vi "Periodic Tasks.vi"(8 "error in":errorcluster) -> ()   [LabVIEW 2016]
doc: "This VI runs in parallel to other tasks. It can contain as many user-defined periodic loops as you need. These can carry out PID or other sorts of timed response."
uses:
  <vilib>/Rock Robotics/WPI/Utilities/WPI_GetSetVariantRefNum.vi
  <vilib>/Rock Robotics/Network Tables/NT Write Number.vi
  <vilib>/Instr/_visa.llb/VISA Configure Serial Port (Instr).vi
  Systems/Global 1.vi
  Global 2.vi
panel:
  in  "Gyro Reset":bool
  out "Angle":dbl
  in  "Reset Drive":bool
  out "Waveform Chart":dbl(graph)
  out "PSI":dbl=101.0986199
  out "Shoot 0":dbl format="%#_13g"
  out "Shoot 1":dbl format="%#_13g"
  out "read buffer":string="B:2,X:203.00"
  in  "Search_Params":string[](array[string])=["B", "X", "Y", "W1", "H1", "W2", "H2"]
  out "Last Complete Message":string="B:2,X:203.00,Y:125.00,W1:11,H1:27,W2:8,H2:25"
  out "length":i32=44
  in  "off set":dbl format="%#_13g"
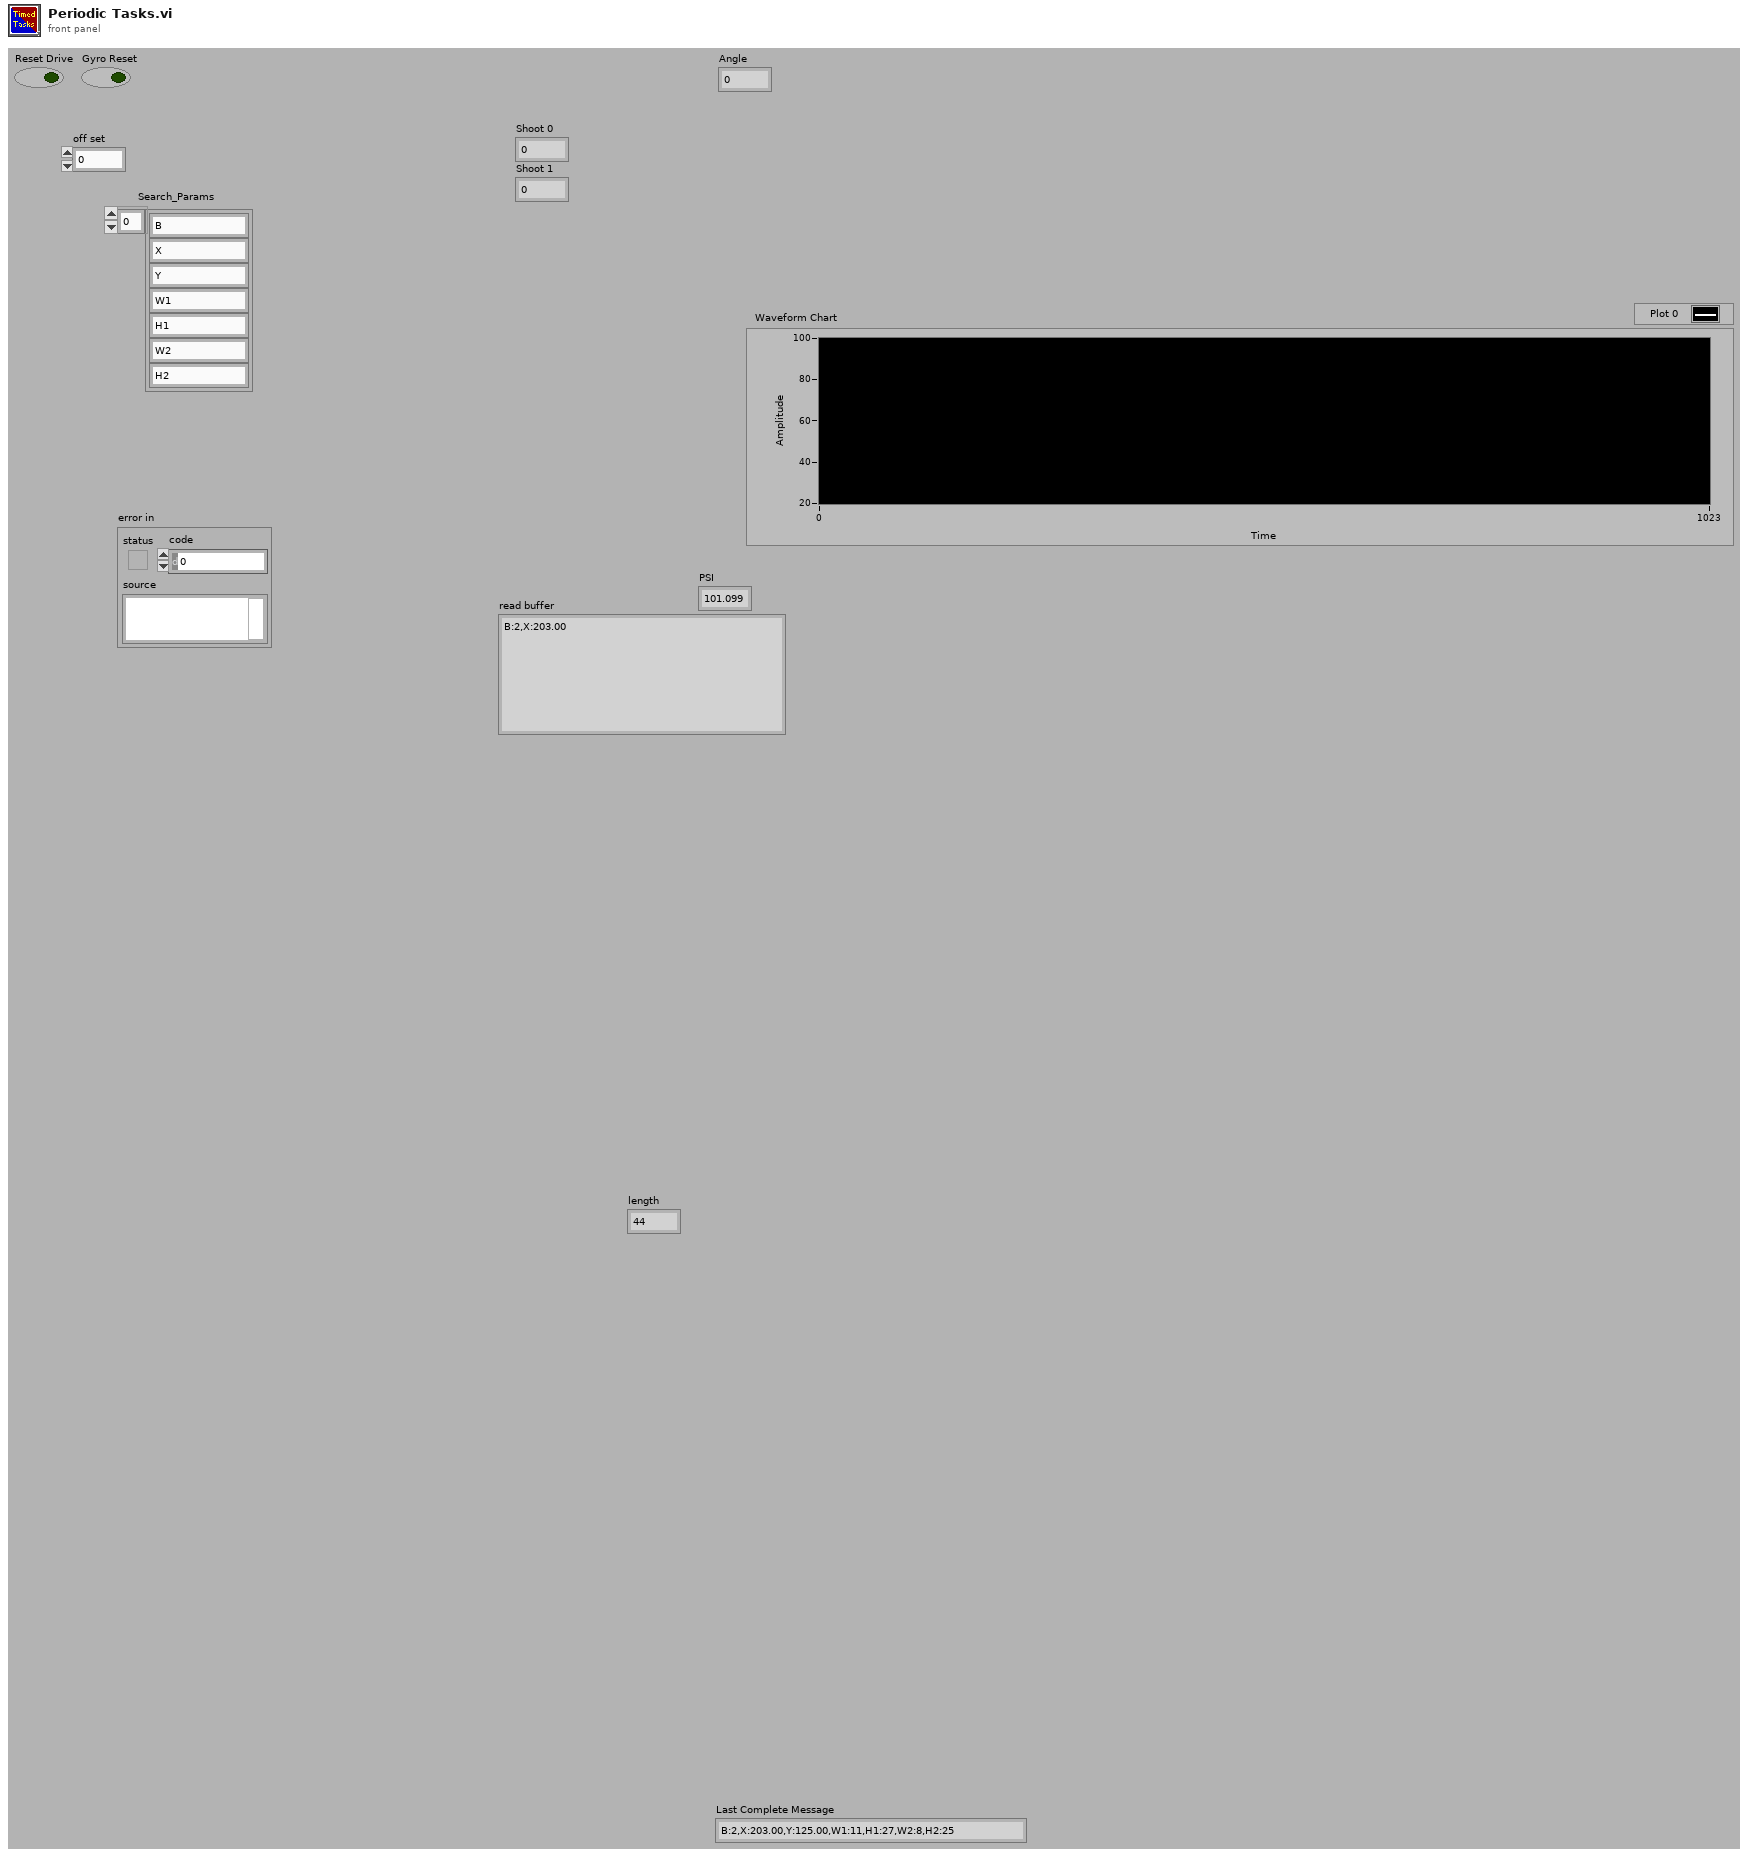
[diagram p1: front panel]
types:
  T1 = typedef "WPI_JoystickDevRef.ctl" = cluster{"Device":T2}
  T2 = typedef "WPI_JoystickDeviceEnum.ctl" = enum16{"USB 0", "USB 1", "USB 2", "USB 3", "USB 4", "USB 5"}
  T3 = typedef "WPI_MotorControlDeviceRef.ctl" = cluster{"DeviceStatus":errorcluster, "Type":T4, "PWM":cluster{"PWM Channel":T5, "DeadBand":T6}, "CAN":cluster{"Device Number":u8, "SetOutput VI Ref":variant, "GetOutput VI Ref":variant, "Enable VI Ref":variant, "Disable VI Ref":variant, "Data":variant}, "Invert":bool}
  T4 = typedef "WPI_MotorControlType.ctl" = enum16{"PWM", "CAN"}
  T5 = typedef "FPGA_DIOPWMChannel.ctl" = enum8{"PWM 0", "PWM 1", "PWM 2", "PWM 3", "PWM 4", "PWM 5", "PWM 6", "PWM 7", "PWM 8", "PWM 9", "PWM MXP 0", "PWM MXP 1", "PWM MXP 2", "PWM MXP 3", "PWM MXP 4", "PWM MXP 5", "PWM MXP 6", "PWM MXP 7", "PWM MXP 8", "PWM MXP 9", "Invalid"}
  T6 = typedef "WPI_PWMDeadband.ctl" = cluster{"Name":string, "maxPositivePwm":i32, "minPositivePwm":i32, "centerPwm":i32, "maxNegativePwm":i32, "minNegativePwm":i32, "angularRange":u16}
  T7 = typedef "WPI_CANTalonSRX_GlobalStatus.ctl" = cluster{"Applied Throttle":dbl, "Module Enabled":bool, "CAN Error":errorcluster, "Closed Loop Error":dbl, "Forward Limit Switch Closed":bool, "Reverse Limit Switch Closed":bool, "Sensor Position":dbl, "Sensor Velocity":dbl, "Current":dbl, "Sticky Fault - Over Temp":bool, "Sticky Fault - Under Voltage":bool, "Sticky Fault - Forward Limit":bool, "Sticky Fault - Reverse Limit":bool, "Sticky Fault - Forward Soft Limit":bool, "Sticky Fault - Reverse Soft Limit":bool, "Brake is Enabled":bool, "Encoder Position":dbl, "Encoder Velocity":dbl, "Encoder Index Count":dbl, "Encoder A Pin State":bool, "Encoder B Pin State":bool, "Encoder Index Pin State":bool, "Analog In":dbl, "Analog In Velocity":dbl, "Temperature (C)":dbl, "Battery Voltage":dbl, "Control 5 Is Supported":bool, "Current Profile Slot Select":dbl, "Pos Div 8":bool, "Vel Div 4":bool, "Pulse Width Position":i32, "Pulse Width Velocity":i32, "Pulse Width Rise To Rise (us)":i32, "Pulse Width Rise To Fall (us)":i32, "Mot Prof Active Is Under Run":bool, "Mot Prof Active Has Under Run":bool, "Mot Prof Active Is Last":bool, "Mot Prof Active Velocity Only":bool, "Mot Prof Active Is Valid":bool, "Mot Prof Buffer Is Full":bool, "Mot Prof Active Profile Slot Select":i32, "Mot Prof NextID":i32, "Mot Prof Count":i32, "Mot Prof Active Velocity":dbl, "Mot Prof Active Position":dbl, "Mot Prof Output Enable":i32}
  T8 = typedef "WPI_AnalogChannelDevRef.ctl" = cluster{"DevStatus":errorcluster, "Analog Channel":T9}
  T9 = typedef "FPGA_AIChannel.ctl" = enum8{"AI 0", "AI 1", "AI 2", "AI 3", "AI MXP 0", "AI MXP 1", "AI MXP 2", "AI MXP 3", "Invalid"}
  T10 = typedef "WPI_GyroDevRef.ctl" = cluster{"DevStatus":errorcluster, "Analog Channel":T9, "Offset":dbl, "Gain (VoltsPerDegree/Second)":dbl, "Gyro Type":enum16{"Analog", "XRS450"}, "Handle":i32, "SPI Bus":T11, "Device Found":bool, "Sample Rate":dbl, "Calibrate On Open":bool}
  T11 = typedef "spi_bus.ctl" = enum16{"SPI On-Board, CS0", "SPI On-Board, CS1", "SPI On-Board, CS2", "SPI On-Board, CS3", "SPI MXP", "Invalid"}
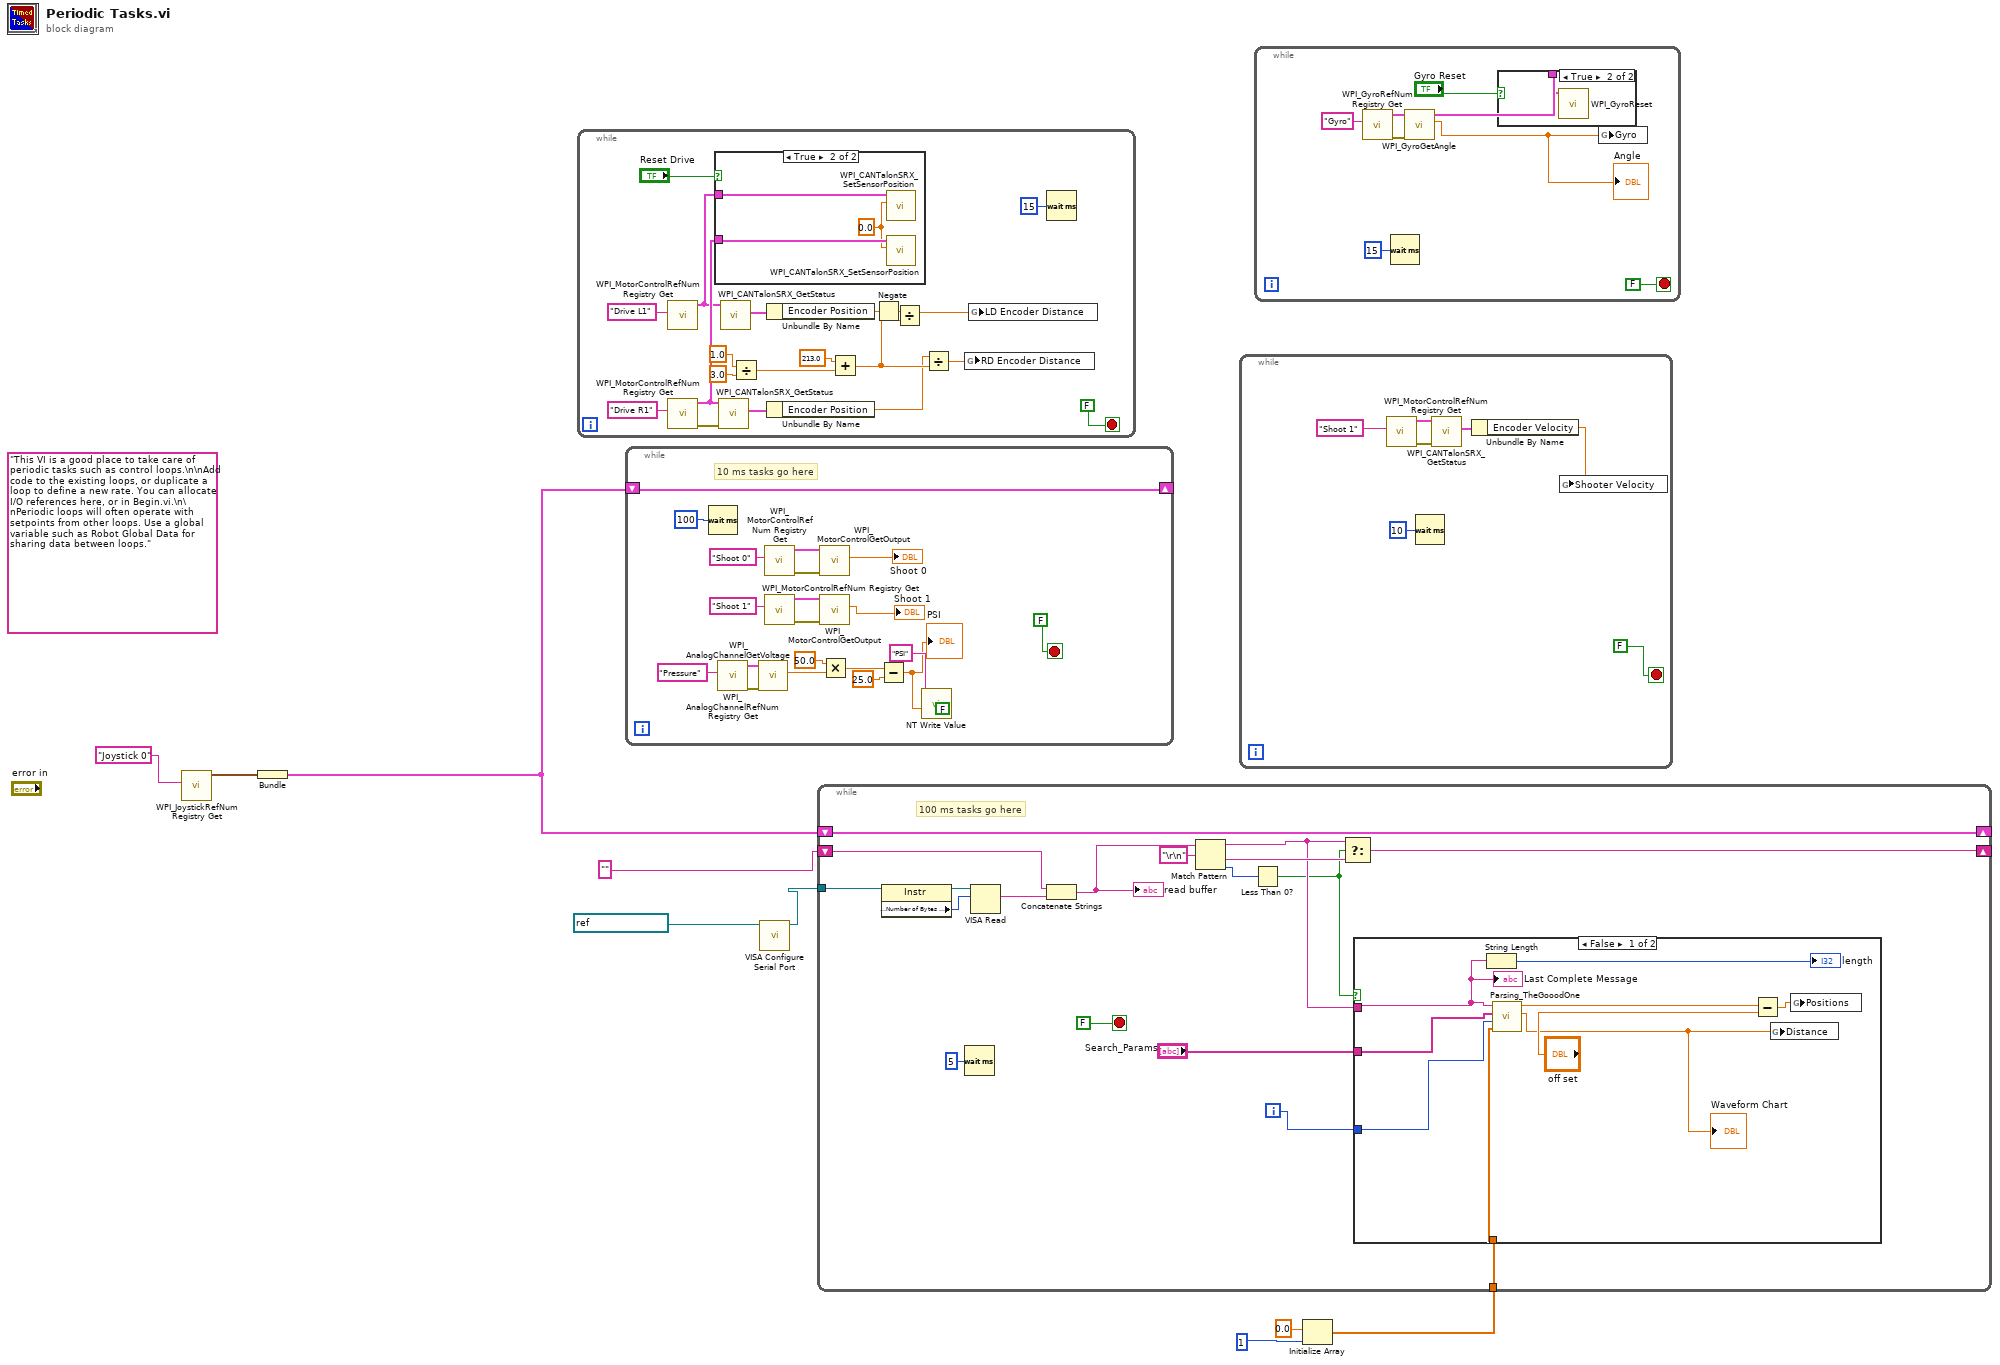
[diagram p0: block diagram]
diagram:
  (unwired) "This VI is a good place to take care of periodic tasks such as control loops.\n\nAdd code to the existing loops, or duplicate a loop to define a new rate. You can allocate I/O references here, or in Begin.vi.\n\nPeriodic loops will often operate with setpoints from other loops. Use a global variable such as Robot Global Data for sharing data between loops."
  n1 = call <vilib>:"WPI_JoystickRefNum Registry Get.vi"("refnum name"="Joystick 0") -> ("JoystickDevRef"=w2:T1)  [unwired: 1 in, 9 out]
  n2 = Bundle("JoystickDevRef"=w2) -> (w3:cluster{"JoystickDevRef":T1})  [unwired: 1 out]
  n3 = while {
    stop <- FALSE stop-if-true
    n4 = call <vilib>:"WPI_MotorControlRefNum Registry Get.vi"("refnum name"="Drive L1") -> ("MotorControlDevRef"=w22:T3)  [unwired: 9 in, 1 out]
    n5 = call <vilib>:"WPI_MotorControlRefNum Registry Get.vi"("refnum name"="Drive R1") -> ("error out"=w27:errorcluster, "MotorControlDevRef"=w23:T3)  [unwired: 9 in]
    n6 = case shown="True" "Reset Drive" {
      tunnel: w23 -> [_ w32]
      tunnel: w22 -> [_ w31]
      frame False {
      }
      frame True {
        w30 = 0.0
        n7 = call <vilib>:"WPI_CANTalonSRX_SetSensorPosition.vi"("New Sensor Position"=w30, "CAN Talon SRX Ref"=w31) -> ()  [unwired: 8 in, 2 out]
        n8 = call <vilib>:"WPI_CANTalonSRX_SetSensorPosition.vi"("New Sensor Position"=w30, "CAN Talon SRX Ref"=w32) -> ()  [unwired: 8 in, 2 out]
      }
    }
    n9 = call <vilib>:"WPI_CANTalonSRX_GetStatus.vi"("error in (no error)"=w27, "CAN Talon SRX Ref"=w23) -> ("Talon SRX Status"=w28:T7)  [unwired: 7 in, 2 out]
    n10 = call <vilib>:"WPI_CANTalonSRX_GetStatus.vi"("CAN Talon SRX Ref"=w22) -> ("Talon SRX Status"=w25:T7)  [unwired: 8 in, 2 out]
    n11 = Divide(x=1.0, y=3.0) -> (x/y=w18:dbl)
    n12 = Unbundle By Name(w25) -> ("Encoder Position"=w16:dbl)
    n13 = Unbundle By Name(w28) -> ("Encoder Position"=w12:dbl)
    n14 = Add(x=213.0, y=w18) -> (x+y=w15:dbl)
    n15 = Negate(x=w16) -> (-x=w10:dbl)
    n16 = Divide(x=w10, y=w15) -> (x/y=w11:dbl)
    n17 = Divide(x=w12, y=w15) -> (x/y=w14:dbl)
    n18 = global write "Global 2.vi" "RD Encoder Distance"(w14) -> ()
    n19 = global write "Global 2.vi" "LD Encoder Distance"(w11) -> ()
    n20 = Wait (ms)(milliseconds to wait=u32 15) -> ()  [unwired: 1 out]
  }
  n21 = while {
    shift-right: [w50] -> _
    shift-left: w3 -> [w50]
    stop <- FALSE stop-if-true
    (unwired) FALSE
    # "10 ms tasks go here"
    n22 = Wait (ms)(milliseconds to wait=u32 100) -> ()  [unwired: 1 out]
    n23 = call <vilib>:"WPI_AnalogChannelRefNum Registry Get.vi"("refnum name"="Pressure") -> ("error out"=w41:errorcluster, "AIDeviceRef"=w40:T8)  [unwired: 9 in]
    n24 = call <vilib>:"WPI_AnalogChannelGetVoltage.vi"("error in (no error)"=w41, "AIDeviceRef"=w40) -> ("Voltage"=w38:dbl)  [unwired: 7 in, 2 out]
    n25 = call <vilib>:"WPI_MotorControlRefNum Registry Get.vi"("refnum name"="Shoot 0") -> ("error out"=w45:errorcluster, "MotorControlDevRef"=w49:T3)  [unwired: 9 in]
    n26 = call <vilib>:"WPI_MotorControlRefNum Registry Get.vi"("refnum name"="Shoot 1") -> ("error out"=w44:errorcluster, "MotorControlDevRef"=w46:T3)  [unwired: 9 in]
    n27 = call <vilib>:"WPI_MotorControlGetOutput.vi"("error in"=w45, "MotorControlDevRef"=w49) -> ("Output"=→"Shoot 0":dbl)  [unwired: 7 in, 2 out]
    n28 = call <vilib>:"WPI_MotorControlGetOutput.vi"("error in"=w44, "MotorControlDevRef"=w46) -> ("Output"=→"Shoot 1":dbl)  [unwired: 7 in, 2 out]
    n29 = Multiply(x=50.0, y=w38) -> (x*y=w36:dbl)
    n30 = Subtract(x=w36, y=25.0) -> (x-y=w33:dbl)
    "PSI" <- w33
    n31 = call-poly <vilib>:"NT Write Value.vi"("Numeric"=w33, "Name"="PSI") -> ()  [unwired: 9 in, 1 out]
  }
  n32 = call-poly "VISA Configure Serial Port"("VISA resource name"=refnum<visa-resource-name> "ASRL2::INSTR") -> ("VISA resource name out"=w5:refnum<visa-resource-name>)  [unwired: 13 in, 1 out]
  n33 = while {
    stop <- FALSE stop-if-true
    n34 = call <vilib>:"WPI_MotorControlRefNum Registry Get.vi"("refnum name"="Shoot 1") -> ("error out"=w57:errorcluster, "MotorControlDevRef"=w58:T3)  [unwired: 9 in]
    n35 = Wait (ms)(milliseconds to wait=u32 10) -> ()  [unwired: 1 out]
    n36 = call <vilib>:"WPI_CANTalonSRX_GetStatus.vi"("error in (no error)"=w57, "CAN Talon SRX Ref"=w58) -> ("Talon SRX Status"=w56:T7)  [unwired: 7 in, 2 out]
    n37 = Unbundle By Name(w56) -> ("Encoder Velocity"=w55:dbl)
    n38 = global write "Global 2.vi" "Shooter Velocity"(w55) -> ()
  }
  n39 = while {
    stop <- FALSE stop-if-true
    n40 = call <vilib>:"WPI_GyroRefNum Registry Get.vi"("refnum name"="Gyro") -> ("error out"=w64:errorcluster, "GyroDevRef"=w67:T10)  [unwired: 9 in]
    n41 = Wait (ms)(milliseconds to wait=u32 15) -> ()  [unwired: 1 out]
    n42 = call <vilib>:"WPI_GyroGetAngle.vi"("error in"=w64, "GyroDevRef"=w67) -> ("Angle"=w61:dbl, "GyroDevRef"=w63:T10)  [unwired: 5 in, 3 out]
    "Angle" <- w61
    n43 = case shown="True" "Gyro Reset" {
      tunnel: w63 -> [_ w68]
      frame False {
      }
      frame True {
        n44 = call <vilib>:"WPI_GyroReset.vi"("GyroDevRef"=w68) -> ()  [unwired: 9 in, 2 out]
      }
    }
    n45 = global write "Global 2.vi" "Gyro"(w61) -> ()
  }
  n46 = Initialize Array(0.0 ("element"), 1) -> (w9:dbl[])
  n47 = while {
    shift-right: [w85] -> _
    shift-left: w3 -> [w85]
    tunnel: w5 -> [w80]
    shift-right: [w72] -> _
    shift-left: "" -> [w79]
    tunnel: w9 -> [w69]
    i -> [w70]
    stop <- FALSE stop-if-true
    # "100 ms tasks go here"
    n48 = property class="Instr"(reference=w80) -> (reference out=w84:refnum<visa-resource-name>, "Serial Settings:Number of Bytes at Serial Port"=w83:u32)  [unwired: 1 in, 1 out]
    n49 = Wait (ms)(milliseconds to wait=u32 5) -> ()  [unwired: 1 out]
    n50 = VISA Read(VISA resource name=w84, byte count=w83) -> (read buffer=w78:string)  [unwired: 1 in, 3 out]
    n51 = Concatenate Strings(w79, w78) -> (w77:string)
    "read buffer" <- w77
    n52 = Match Pattern(string=w77, regular expression="\r\n") -> (before substring=w73:string, after substring=w74:string, offset past match=w75:i32)  [unwired: 1 in, 1 out]
    n53 = Less Than 0?(x=w75) -> (x < 0?=w71:bool)
    n54 = Select(t=w73, s=w71, f=w74) -> (s? t:f=w72:string)
    n55 = case shown="False" w71 {
      tunnel: "Search_Params" -> [w94 _]
      tunnel: w73 -> [w93 _]
      tunnel: w70 -> [w89 _]
      tunnel: w69 -> [w88 _]
      frame False {
        n56 = String Length(string=w93) -> (length=→"length":i32)
        n57 = call "Parsing_TheGooodOne.vi"("array"=w88, "Iterations"=w89, "Search_Params"=w94, "Input"=w93) -> ("Corrected distance"=w87:dbl, "Value-Reference"=w92:dbl)  [unwired: 4 in]
        "Waveform Chart" <- w87
        n58 = Subtract(x=w92, y="off set") -> (x-y=w90:dbl)
        n59 = global write "Global 1.vi" "Distance"(w87) -> ()
        n60 = global write "Global 1.vi" "Positions"(w90) -> ()
        "Last Complete Message" <- w93
      }
      frame True {
      }
    }
  }
